vi "List Directory and LLBs.vi"(6 "pattern":string, 8 "error in (no error)":errorcluster, 11 "Folder Path":path) -> (0 "error out":errorcluster, 1 "Folders and LLBs":string[](array[string]), 2 "Files sans LLBs":string[](array[string]), 3 "dup Folder Path":path)   [LabVIEW 2014]
doc: "This VI acts like the \"List Directory\" function, but treats LLBs as folders.\n\nNote: In order for this VI to work properly, your LLBs must have a .llb extension."
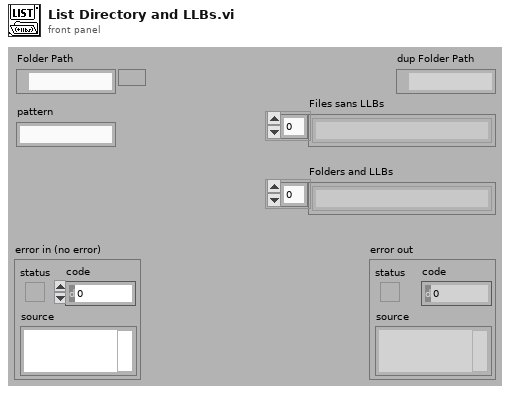
[diagram p1: front panel]
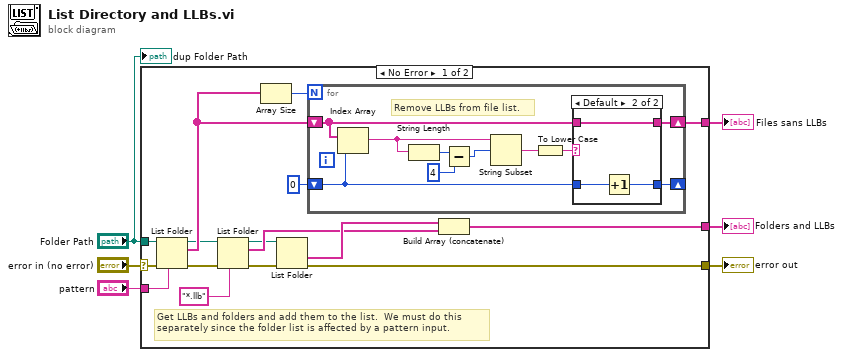
[diagram p0: block diagram]
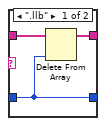
[diagram p2: hidden frame]
diagram:
  n1 = case shown="No Error" "error in (no error)" {
    selector: "error in (no error)" -> [w17 w39]
    tunnel: [w22 _] -> w6
    tunnel: "Folder Path" -> [w21 _]
    tunnel: [w11 w39] -> w4
    tunnel: [w8 _] -> w2
    tunnel: "pattern" -> [w16 _]
    frame No Error {
      # "Get LLBs and folders and add them to the list.  We must do this\nseparately since the folder list is affected by a pattern input."
      n2 = List Folder(path=w21, pattern=w16, error in=w17) -> (path out=w14:path, filenames=w18:string[], error out=w15:errorcluster)  [unwired: 2 out]
      n3 = List Folder(path=w14, pattern="*.llb", error in=w15) -> (path out=w7:path, filenames=w9:string[], error out=w12:errorcluster)  [unwired: 2 out]
      n4 = Array Size(array=w18) -> (size(s)=w19:i32)
      n5 = List Folder(path=w7, error in=w12) -> (folder names=w10:string[], error out=w11:errorcluster)  [unwired: 4 out]
      n6 = for {
        N: w19 -> [_]
        shift-right: [w31] -> w22
        shift-left: w18 -> [w32]
        shift-right: [w29] -> _
        shift-left: 0 -> [w30]
        # "Remove LLBs from file list."
        n7 = Index Array(array=w32, index=w30) -> (element=w23:string)
        n8 = String Length(string=w23) -> (length=w28:i32)
        n9 = Subtract(x=w28, y=4) -> (x-y=w26:i32)
        n10 = String Subset(string=w23, offset (0)=w26) -> (substring=w24:string)  [unwired: 1 out]
        n11 = To Lower Case(string=w24) -> (all lower case string=w25:string)
        n12 = case shown="Default" w25 {
          tunnel: w32 -> [w35 w36]
          tunnel: w30 -> [w34 w38]
          tunnel: [w34 w37] -> w29
          tunnel: [w33 w36] -> w31
          frame ".llb" {
            n13 = Delete From Array(array=w35, index=w34) -> (array with subset deleted=w33:string[])  [unwired: 1 in, 1 out]
          }
          frame Default {
            n14 = Increment(x=w38) -> (x+1=w37:i32)
          }
        }
      }
      n15 = Build Array (concatenate)(w10, w9) -> (w8:string[])
    }
    frame Error {
    }
  }
  "Files sans LLBs" <- w6
  "error out" <- w4
  "Folders and LLBs" <- w2
  "dup Folder Path" <- "Folder Path"
